vi "Call Functions.vi"(11 "Data In":string) -> (3 "Data Out":string)   [LabVIEW 2018, in "Labview Python.lvlib"]
uses:
  Labview Python.lvlib
panel:
  in  "Cluster":cluster{"Command":string, "Data":string}
  out "Data":string
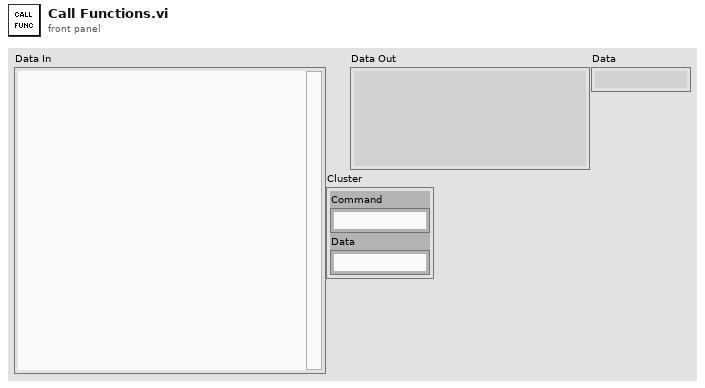
[diagram p1: front panel]
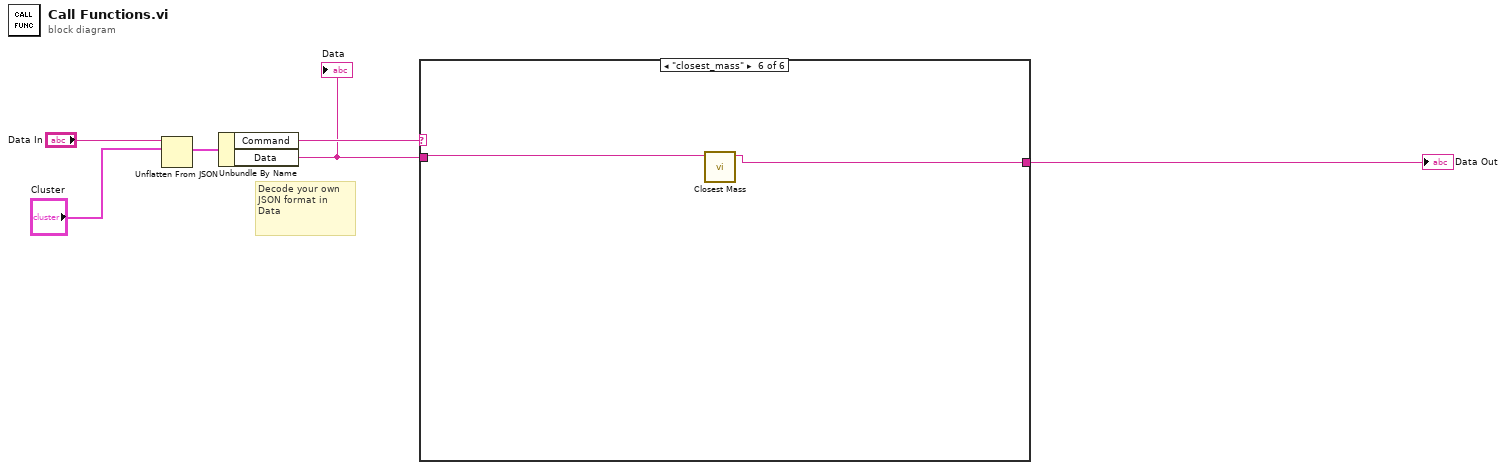
[diagram p0: block diagram]
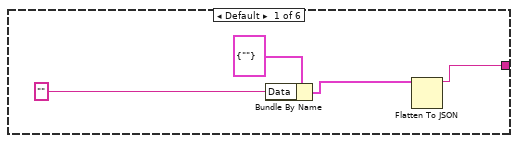
[diagram p2: hidden frame]
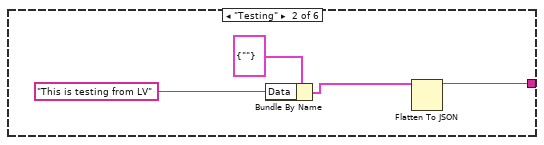
[diagram p3: hidden frame]
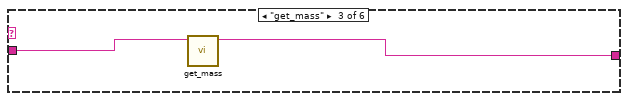
[diagram p4: hidden frame]
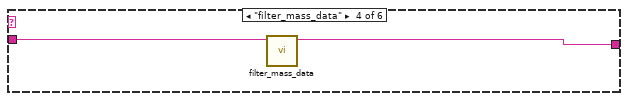
[diagram p5: hidden frame]
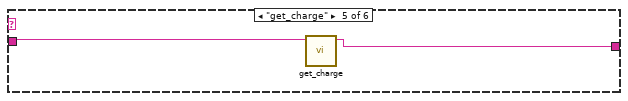
[diagram p6: hidden frame]
diagram:
  # "Decode your own JSON format in Data"
  n1 = Unflatten From JSON(JSON string="Data In", type and defaults="Cluster") -> (value=w5:cluster{"Command":string, "Data":string})  [unwired: 5 in, 1 out]
  n2 = Unbundle By Name(w5) -> ("Command"=w4:string, "Data"=w3:string)
  "Data" <- w3
  n3 = case shown="\"closest_mass\"" w4 {
    tunnel: w3 -> [_ _ w16 w18 w20 w22]
    tunnel: [w7 w12 w15 w17 w19 w21] -> w1
    frame Default {
      n4 = Bundle By Name(cluster=cluster{"Data":string} {"Data"=""} ("Cluster 2"), "Data"="") -> (w9:cluster{"Data":string})
      n5 = Flatten To JSON(anything=w9) -> (JSON string=w7:string)  [unwired: 2 in, 1 out]
    }
    frame "Testing" {
      n6 = Bundle By Name(cluster=cluster{"Data":string} {"Data"=""} ("Cluster 2"), "Data"="This is testing from LV") -> (w11:cluster{"Data":string})
      n7 = Flatten To JSON(anything=w11) -> (JSON string=w12:string)  [unwired: 2 in, 1 out]
    }
    frame "get_mass" {
      n8 = call "get_mass.vi"("Data In"=w16) -> ("Data Out"=w15:string)  [unwired: 10 in]
    }
    frame "filter_mass_data" {
      n9 = call "filter_mass_data.vi"("Data In"=w18) -> ("Data Out"=w17:string)  [unwired: 10 in]
    }
    frame "get_charge" {
      n10 = call "get_charge.vi"("Data In"=w20) -> ("Data Out"=w19:string)  [unwired: 10 in]
    }
    frame "closest_mass" {
      n11 = call "Closest Mass.vi"("Data In"=w22) -> ("Data Out"=w21:string)  [unwired: 10 in]
    }
  }
  "Data Out" <- w1
